vi "Lex & Unescaped Variable.vi"(8 "Error In":errorcluster) -> (0 "Error Out":errorcluster)   [LabVIEW 2018, in "Tests.lvlib" / "Lexer.lvlib"]
uses:
  Lexer.lvlib
  src/Toolkit/Low-Level/Tokens/UnescapedVariable/UnescapedVariable.lvclass
  src/Toolkit/Low-Level/Tokens/Keyable/Keyable.lvclass/Keyable.ctl
  src/Toolkit/Low-Level/Tokens/Keyable/Read Key.vi
  src/Toolkit/Low-Level/Support/Lex String.vi
  <vilib>/Utility/LVClass/Get LV Class Name.vi
  src/Toolkit/Low-Level/Tokens/Keyable/Keyable.lvclass
  <vilib>/addons/_JKI Toolkits/Caraya/classes/Test/Test.lvclass
  <vilib>/addons/_JKI Toolkits/Caraya/classes/Assert/Assert.lvclass
  Tests.lvlib
  src/Toolkit/Toolkit.lvlib
  src/Toolkit/Low-Level/Tokens/Abstract/Abstract.lvclass
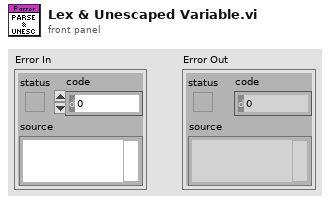
[diagram p1: front panel]
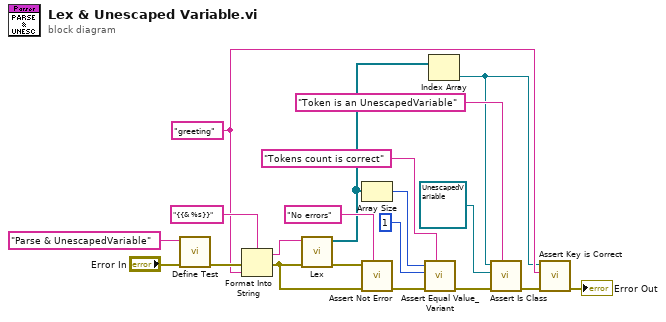
[diagram p0: block diagram]
diagram:
  w5 = "greeting"
  n1 = call <vilib>:"Define Test.vi"("error in (no error)"="Error In", "Label (VI Title)"="Parse & UnescapedVariable") -> ("error out"=w17:errorcluster)  [unwired: 9 in]
  n2 = Format Into String(format string="{{& %s}}", error in=w17, w5) -> (resulting string=w2:string, error out=w1:errorcluster)  [unwired: 1 in]
  n3 = call-poly "Lex.vi"("Error In"=w1, "Input"=w2) -> ("Error Out"=w18:errorcluster, "Tokens"=w11:refnum<class "Abstract.lvclass">[])  [unwired: 8 in]
  n4 = Array Size(array=w11) -> (size(s)=w13:i32)
  n5 = call <vilib>:"Assert Not Error.vi"("Label"="No errors", "error in (no error)"=w1, "Not Error?"=w18) -> ("error out"=w15:errorcluster)  [unwired: 8 in]
  n6 = call <vilib>:"Assert Equal Value_Variant.vi"("Label"="Tokens count is correct", "error in (no error)"=w15, "Y"=1 ("size(s)"), "X"=w13) -> ("error out"=w10:errorcluster)  [unwired: 7 in]
  n7 = Index Array(array=w11) -> (element=w4:refnum<class "Abstract.lvclass">)  [unwired: 1 in]
  n8 = call "Assert Is Class.vi"("Label"="Token is an UnescapedVariable", "Error In"=w10, "Expected"=refnum<class "UnescapedVariable.lvclass"> refnum ("Mustache.lvlib:Tokens.lvlib:UnescapedVariable.lvclass"), "Actual"=w4) -> ("Error Out"=w3:errorcluster)  [unwired: 7 in]
  n9 = call "Assert Key is Correct.vi"("Error In"=w3, "Expected"=w5, "Token"=w4) -> ("Error Out"=→"Error Out":errorcluster)  [unwired: 8 in]
